vi "Init Color.vi"(8 "error in (no error)":errorcluster, 11 "Terminal in":refnum<class "Terminal.lvclass">) -> (0 "error out":errorcluster, 3 "Terminal out":refnum<class "Terminal.lvclass">)   [LabVIEW 2020, in "Terminal.lvlib" / "Terminal.lvclass"]
uses:
  Terminal.lvclass
  Terminal.lvclass/Terminal.ctl
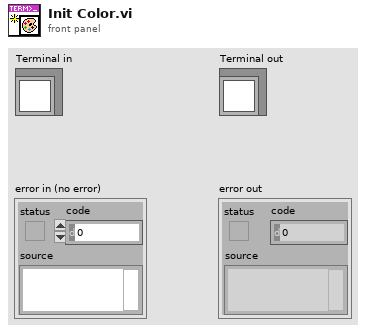
[diagram p1: front panel]
types:
  T1 = typedef "Terminal.lvlib/Terminal.lvclass/Ref Data.ctl" = cluster{"Connection":refnum<class "Connection.lvclass">, "Read Loop Running":bool, "Parse State":T2, "Terminal Options":T3}
  T2 = typedef "Terminal.lvlib/Terminal.lvclass/Parse State.ctl" = cluster{"Sequence":string, "ESC":bool, "CSI":bool, "DCS":bool, "OSC":bool, "Cur Row":i32, "Cur Col":i32, "Saved Row":i32, "Saved Col":i32, "FG":u32, "BG":u32, "Bold":bool, "Italic":bool, "Underline":bool, "Strike":bool, "Inverse":bool}
  T3 = typedef "Terminal.lvlib/Terminal Options.ctl" = cluster{"Implied CR with LF":bool, "Local Echo":bool, "Tab Width":i32, "Color Scheme":T4, "Default FG":T5, "Default BG":T5, "History Length":i32, "Font Face":string, "Font Size":i16}
  T4 = typedef "Terminal.lvlib/Color Scheme.ctl" = cluster{"Black":u32, "Red":u32, "Green":u32, "Yellow":u32, "Blue":u32, "Magenta":u32, "Cyan":u32, "White":u32, "Bright Black":u32, "Bright Red":u32, "Bright Green":u32, "Bright Yellow":u32, "Bright Blue":u32, "Bright Magenta":u32, "Bright Cyan":u32, "Bright White":u32}
  T5 = typedef "Terminal.lvlib/Color.ctl" = i8
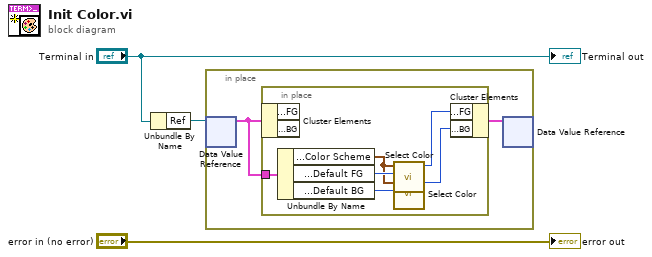
[diagram p0: block diagram]
diagram:
  n1 = Unbundle By Name("Terminal in") -> ("Ref"=w2:refnum<data-value>)
  n2 = in-place {
    n3 = in-place-dvr #1(w2) -> (w4:T1)  [unwired: 1 out]
    n4 = in-place {
      in-place-border: w4 -> [w11]
      n5 = in-place-cluster #2(w4) -> ()  [unwired: 2 out]
      n6 = Unbundle By Name(w11) -> ("Terminal Options.Color Scheme"=w8:T4, "Terminal Options.Default FG"=w10:T5, "Terminal Options.Default BG"=w9:T5)
      n7 = call "Select Color.vi"("Color"=w10, "Color Scheme"=w8) -> ("Color Value"=w7:u32)  [unwired: 9 in]
      n8 = call "Select Color.vi"("Color"=w9, "Color Scheme"=w8) -> ("Color Value"=w6:u32)  [unwired: 9 in]
      n9 = in-place-cluster #2("Parse State.FG"=w7, "Parse State.BG"=w6) -> (w5:T1)
    }
    n10 = in-place-dvr #1(w5) -> ()  [unwired: 2 out]
  }
  "error out" <- "error in (no error)"
  "Terminal out" <- "Terminal in"
